vi "Menu Act Show Context Help.vi"(8 "error in (no error)":errorcluster, 11 "LF2R IDE in":refnum<class "LF2R IDE.lvclass">) -> (0 "error out":errorcluster, 3 "LF2R IDE out":refnum<class "LF2R IDE.lvclass">)   [LabVIEW 2018, in "LF2R IDE.lvlib" / "LF2R IDE.lvclass"]
uses:
  LF2R IDE.lvclass
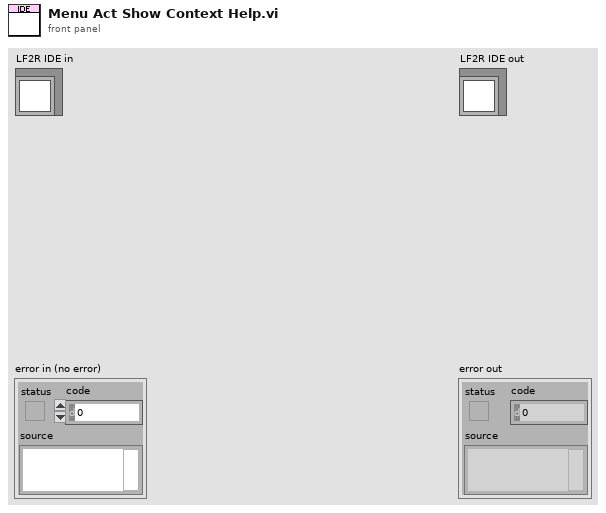
[diagram p1: front panel]
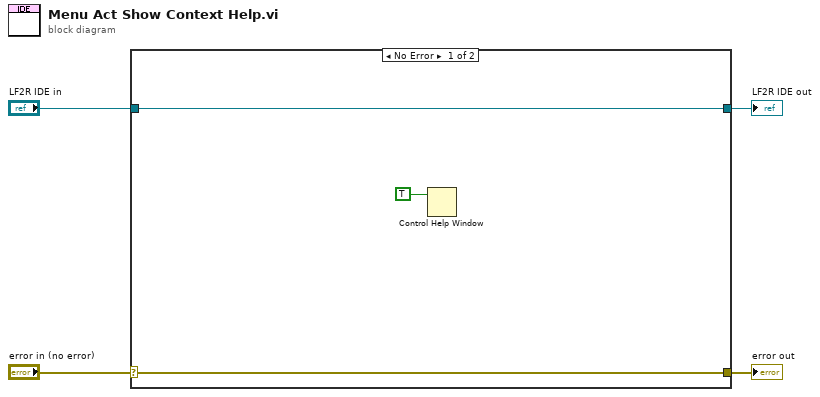
[diagram p0: block diagram]
diagram:
  n1 = case shown="No Error" "error in (no error)" {
    selector: "error in (no error)" -> [w7 w9]
    tunnel: [w7 w9] -> w3
    tunnel: [w6 w8] -> w1
    tunnel: "LF2R IDE in" -> [w6 w8]
    frame No Error {
      n2 = Control Help Window(1:TRUE ("Show")) -> ()  [unwired: 1 in]
    }
    frame Error {
    }
  }
  "error out" <- w3
  "LF2R IDE out" <- w1
